vi "Projet_Rachdaoui_Bollard.vi"() -> ()   [LabVIEW 2019]
uses:
  <vilib>/Platform/TimedLoop/XDataNode/timing_clust.ctl
  <vilib>/Platform/TimedLoop/XDataNode/nitl_modes.ctl
  <vilib>/Platform/TimedLoop/XDataNode/wakeup.ctl
  <vilib>/rvi/eio/common/nirviEmuTemplateMethod_errors.vi
  <vilib>/rvi/Emulation/niFpgaSctlEmulationGetInTimedLoop.vi
  <vilib>/rvi/Emulation/niFpgaEmulationReportErrorSimple.vi
  <vilib>/rvi/Emulation/niFpgaGetClockAttributes.vi
  <vilib>/rvi/Emulation/niFpgaCriticalErrorInLSC.vi
  <vilib>/eio/EIONode/EIONode.xnode
  <vilib>/eio/EIOMethodNode/EIOMethodNode.xnode
  <vilib>/platform/TimedLoop/XDataNode/XDataNode.xnode
  <vilib>/Platform/TimedLoop/XDataNode/XDNodeRunTimeDep.lvlib
panel:
  out "SDA":bool
  in  "Address device + read":i16=51
  out "Address device + write":bool[](array[boolean])
  out "Register":bool[](array[boolean])
  out "Dumy register":bool[](array[boolean])
  in  "Register":i16=15
  in  "Address device + write":i16=50
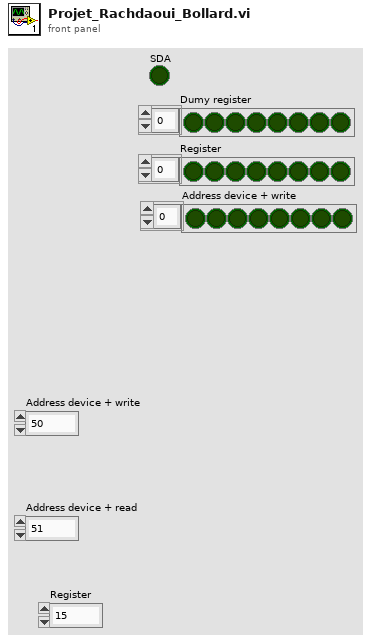
[diagram p1: front panel]
types:
  T1 = typedef "XDNodeRunTimeDep.lvlib/timing_clust.ctl" = cluster{"Expected End [f-1]":u64, "Actual End [f-1]":u64, "Finished Late? [f-1]":bool, "Expected End [i-1]":u64, "Actual End [i-1]":u64, "Finished Late? [i-1]":bool, "Expected Start [i]":u64, "Actual Start [i]":u64, "Expected Start [f]":u64, "Actual Start [f]":u64, "Source Name":string, "Structure Name":string, "Period":i64, "Deadline":i64, "Offset":i64, "Start":i64, "Priority":i32, "Timeout":i32, "Mode":T2, "Wakeup Reason":T3, "Error":errorcluster, "Source Type":string, "Secondary Source Type":string, "Global End Time":u64, "Global Start Time":u64, "Frame Duration":u64, "Iteration Duration":u64, "Assigned CPU":i32, "I/O Scan Engine Mode":u32}
  T2 = typedef "XDNodeRunTimeDep.lvlib/nitl_modes.ctl" = enum32{"No Change", "Process missed periods, maintain original phase", "Discard missed periods, maintain original phase", "Process missed periods, ignore original phase", "Discard missed periods, ignore original phase"}
  T3 = typedef "XDNodeRunTimeDep.lvlib/wakeup.ctl" = enum32{"Normal", "Aborted", "Asynchronous wakeup", "Timing source error", "Timed loop error", "Timeout"}
diagram:
  n1 = flat-sequence {
    frame #0 {
      # "start condition"
      n2 = xnode "FPGA I/O Node"("CLK"=TRUE) -> ()  [unwired: 1 in, 1 out]
      n3 = xnode "FPGA I/O Node"("SDA"=TRUE) -> ()  [unwired: 1 in, 1 out]
    }
    frame #1 {
      n4 = call "Wait2"("Count(Ticks)"=u16 500) -> ()  [unwired: 1 out]
    }
    frame #2 {
      # "start condition"
      n5 = xnode "FPGA I/O Node"("SDA"=FALSE) -> ()  [unwired: 1 in, 1 out]
    }
    frame #3 {
      n6 = call "Wait16"("Count(Ticks)"=u16 500) -> ()  [unwired: 1 out]
    }
    frame #4 {
      n7 = xnode "FPGA I/O Node"("CLK"=FALSE) -> ()  [unwired: 1 in, 1 out]
    }
    frame #5 {
      # "Device address"
      n8 = Number To Boolean Array(number="Address device + write") -> (Boolean array=w8:bool[])
      "Address device + write" <- w8
      n9 = for {
        N: 8 -> [_]
        tunnel: w8 -> [w10] mode=indexing
        n10 = flat-sequence {
          tunnel: w10 -> [w11]
          frame #0 {
            n11 = xnode "FPGA I/O Node"("SDA"=w11) -> ()  [unwired: 1 in, 1 out]
          }
          frame #1 {
            n12 = call "Wait3"("Count(Ticks)"=u16 500) -> ()  [unwired: 1 out]
          }
          frame #2 {
            n13 = xnode "FPGA I/O Node"("CLK"=TRUE) -> ()  [unwired: 1 in, 1 out]
          }
          frame #3 {
            n14 = call "Wait15"("Count(Ticks)"=u16 500) -> ()  [unwired: 1 out]
          }
          frame #4 {
            n15 = xnode "FPGA I/O Node"("CLK"=FALSE) -> ()  [unwired: 1 in, 1 out]
          }
        }
      }
    }
    frame #6 {
      n16 = xnode "FPGA I/O Node"("CLK"=FALSE) -> ()  [unwired: 1 in, 1 out]
      n17 = xnode "FPGA I/O Method Node"("Enable"=FALSE) -> ()  [unwired: 1 in, 1 out]
    }
    frame #7 {
      n18 = call "Wait11"("Count(Ticks)"=u16 500) -> ()  [unwired: 1 out]
    }
    frame #8 {
      # "Aknowledge"
      n19 = node-c288() -> (w20:T1)  [unwired: 1 in]
      n20 = timed-loop {
        timing: w20 -> [_]
        timing-out: [_] -> w19
        stop <- w21 stop-if-true
        n21 = xnode "FPGA I/O Node"() -> ("SDA"=w21:bool)  [unwired: 1 in, 1 out]
      }
      n22 = node-c288(w19) -> ()
    }
    frame #9 {
      n23 = call "Wait12"("Count(Ticks)"=u16 500) -> ()  [unwired: 1 out]
    }
    frame #10 {
      # "Register adress"
      n24 = Number To Boolean Array(number="Register") -> (Boolean array=w27:bool[])
      "Register" <- w27
      n25 = for {
        N: 8 -> [_]
        tunnel: w27 -> [w30] mode=indexing
        n26 = flat-sequence {
          tunnel: w30 -> [w31]
          frame #0 {
            n27 = xnode "FPGA I/O Node"("SDA"=w31) -> ()  [unwired: 1 in, 1 out]
          }
          frame #1 {
            n28 = call "Wait17"("Count(Ticks)"=u16 500) -> ()  [unwired: 1 out]
          }
          frame #2 {
            n29 = xnode "FPGA I/O Node"("CLK"=TRUE) -> ()  [unwired: 1 in, 1 out]
          }
          frame #3 {
            n30 = call "Wait18"("Count(Ticks)"=u16 500) -> ()  [unwired: 1 out]
          }
          frame #4 {
            n31 = xnode "FPGA I/O Node"("CLK"=FALSE) -> ()  [unwired: 1 in, 1 out]
          }
        }
      }
    }
    frame #11 {
      n32 = xnode "FPGA I/O Node"("CLK"=FALSE) -> ()  [unwired: 1 in, 1 out]
      n33 = xnode "FPGA I/O Method Node"("Enable"=FALSE) -> ()  [unwired: 1 in, 1 out]
    }
    frame #12 {
      n34 = call "Wait9"("Count(Ticks)"=u16 500) -> ()  [unwired: 1 out]
    }
    frame #13 {
      n35 = xnode "FPGA I/O Node"("CLK"=TRUE) -> ()  [unwired: 1 in, 1 out]
    }
    frame #14 {
      n36 = xnode "FPGA I/O Node"() -> ("SDA"=→"SDA":bool)  [unwired: 1 in, 1 out]
    }
    frame #15 {
      # "aknowledge"
      n37 = node-c288() -> (w42:T1)  [unwired: 1 in]
      n38 = timed-loop {
        timing: w42 -> [_]
        timing-out: [_] -> w41
        stop <- w43 stop-if-true
        n39 = xnode "FPGA I/O Node"() -> ("SDA"=w43:bool)  [unwired: 1 in, 1 out]
      }
      n40 = node-c288(w41) -> ()
    }
    frame #16 {
      n41 = call "Wait10"("Count(Ticks)"=u16 500) -> ()  [unwired: 1 out]
    }
    frame #17 {
    }
    frame #18 {
    }
    frame #19 {
    }
    frame #20 {
    }
    frame #21 {
      # "start condition"
      n42 = xnode "FPGA I/O Node"("CLK"=TRUE) -> ()  [unwired: 1 in, 1 out]
      n43 = xnode "FPGA I/O Node"("SDA"=TRUE) -> ()  [unwired: 1 in, 1 out]
    }
    frame #22 {
      n44 = call "Wait6"("Count(Ticks)"=u16 500) -> ()  [unwired: 1 out]
    }
    frame #23 {
      # "start condition"
      n45 = xnode "FPGA I/O Node"("SDA"=FALSE) -> ()  [unwired: 1 in, 1 out]
    }
    frame #24 {
      n46 = call "Wait13"("Count(Ticks)"=u16 500) -> ()  [unwired: 1 out]
    }
    frame #25 {
      n47 = xnode "FPGA I/O Node"("CLK"=FALSE) -> ()  [unwired: 1 in, 1 out]
    }
    frame #26 {
      # "Device adress + read bit"
      n48 = Number To Boolean Array(number="Address device + read") -> (Boolean array=w55:bool[])
      n49 = for {
        N: 8 -> [_]
        tunnel: w55 -> [w58] mode=indexing
        n50 = flat-sequence {
          tunnel: w58 -> [w59]
          frame #0 {
            n51 = xnode "FPGA I/O Node"("SDA"=w59) -> ()  [unwired: 1 in, 1 out]
          }
          frame #1 {
            n52 = call "Wait"("Count(Ticks)"=u16 500) -> ()  [unwired: 1 out]
          }
          frame #2 {
            n53 = xnode "FPGA I/O Node"("CLK"=TRUE) -> ()  [unwired: 1 in, 1 out]
          }
          frame #3 {
            n54 = call "Wait19"("Count(Ticks)"=u16 500) -> ()  [unwired: 1 out]
          }
          frame #4 {
            n55 = xnode "FPGA I/O Node"("CLK"=FALSE) -> ()  [unwired: 1 in, 1 out]
          }
        }
      }
    }
    frame #27 {
      n56 = xnode "FPGA I/O Method Node"("Enable"=FALSE) -> ()  [unwired: 1 in, 1 out]
      n57 = xnode "FPGA I/O Node"("CLK"=FALSE) -> ()  [unwired: 1 in, 1 out]
    }
    frame #28 {
      n58 = call "Wait14"("Count(Ticks)"=u16 500) -> ()  [unwired: 1 out]
    }
    frame #29 {
      n59 = xnode "FPGA I/O Node"("CLK"=TRUE) -> ()  [unwired: 1 in, 1 out]
    }
    frame #30 {
    }
    frame #31 {
      # "aknowledge"
      n60 = node-c288() -> (w69:T1)  [unwired: 1 in]
      n61 = timed-loop {
        timing: w69 -> [_]
        timing-out: [_] -> w68
        stop <- w70 stop-if-true
        n62 = xnode "FPGA I/O Node"() -> ("SDA"=w70:bool)  [unwired: 1 in, 1 out]
      }
      n63 = node-c288(w68) -> ()
    }
    frame #32 {
      n64 = xnode "FPGA I/O Method Node"("Enable"=FALSE) -> ()  [unwired: 1 in, 1 out]
    }
    frame #33 {
      # "Read data"
      n65 = for {
        N: 8 -> [_]
        tunnel: [w78] -> w76 mode=indexing
        n66 = flat-sequence {
          tunnel: [w82] -> w78
          frame #0 {
            n67 = xnode "FPGA I/O Node"("CLK"=TRUE) -> ()  [unwired: 1 in, 1 out]
          }
          frame #1 {
            n68 = call "Wait7"("Count(Ticks)"=u16 500) -> ()  [unwired: 1 out]
          }
          frame #2 {
            n69 = xnode "FPGA I/O Node"() -> ("SDA"=w82:bool)  [unwired: 1 in, 1 out]
          }
          frame #3 {
            n70 = call "Wait20"("Count(Ticks)"=u16 500) -> ()  [unwired: 1 out]
          }
          frame #4 {
            n71 = xnode "FPGA I/O Node"("CLK"=FALSE) -> ()  [unwired: 1 in, 1 out]
          }
        }
        n72 = call "Wait22"("Count(Ticks)"=u16 500) -> ()  [unwired: 1 out]
      }
      "Dumy register" <- w76
    }
    frame #34 {
      # "NACK"
      n73 = xnode "FPGA I/O Method Node"("Enable"=TRUE) -> ()  [unwired: 1 in, 1 out]
    }
    frame #35 {
      n74 = node-c288() -> (w87:T1)  [unwired: 1 in]
      n75 = timed-loop {
        timing: w87 -> [_]
        timing-out: [_] -> w86
        stop <- w88 stop-if-true
        n76 = xnode "FPGA I/O Node"() -> ("SDA"=w88:bool)  [unwired: 1 in, 1 out]
      }
      n77 = node-c288(w86) -> ()
    }
    frame #36 {
      n78 = call "Wait4"("Count(Ticks)"=u16 500) -> ()  [unwired: 1 out]
    }
    frame #37 {
      # "stop condition"
      n79 = xnode "FPGA I/O Node"("CLK"=FALSE) -> ()  [unwired: 1 in, 1 out]
    }
    frame #38 {
      n80 = call "Wait5"("Count(Ticks)"=u16 500) -> ()  [unwired: 1 out]
    }
    frame #39 {
      # "stop condition"
      n81 = xnode "FPGA I/O Node"("SDA"=TRUE) -> ()  [unwired: 1 in, 1 out]
    }
  }
